vi "Spin In Circles Test (Test Turning PID).vi"() -> ()   [LabVIEW 2017]
uses:
  <vilib>/Platform/TimedLoop/XDataNode/XDataNode.xnode
  <vilib>/Platform/TimedLoop/XDataNode/nitl_modes.ctl
  <vilib>/Platform/TimedLoop/XDataNode/XDNodeRunTimeDep.lvlib
  <vilib>/Platform/TimedLoop/XDataNode/wakeup.ctl
  <vilib>/Platform/TimedLoop/XDataNode/timing_clust.ctl
  Globals/Pose.vi
  Globals/Motor Speed Multiplier.vi
panel:
  in  "Stop motors":bool=TRUE
  in  "Speed":T1={"\nMoving speed"=3.0889830508474576, "Turning speed limit"=1.0677966101694916} {"Turning speed limit" scale=0.0..4.0; "Moving speed" scale=0.0..1.0}
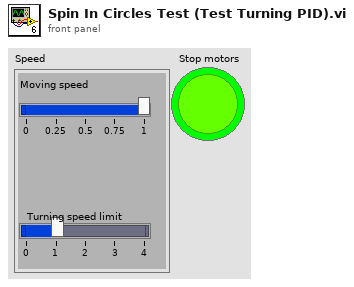
[diagram p1: front panel]
types:
  T1 = cluster{"\nMoving speed":dbl, "Turning speed limit":dbl}
  T2 = typedef "XDNodeRunTimeDep.lvlib/timing_clust.ctl" = cluster{"Expected End [f-1]":u64, "Actual End [f-1]":u64, "Finished Late? [f-1]":bool, "Expected End [i-1]":u64, "Actual End [i-1]":u64, "Finished Late? [i-1]":bool, "Expected Start [i]":u64, "Actual Start [i]":u64, "Expected Start [f]":u64, "Actual Start [f]":u64, "Source Name":string, "Structure Name":string, "Period":i64, "Deadline":i64, "Offset":i64, "Start":i64, "Priority":i32, "Timeout":i32, "Mode":T3, "Wakeup Reason":T4, "Error":errorcluster, "Source Type":string, "Secondary Source Type":string, "Global End Time":u64, "Global Start Time":u64, "Frame Duration":u64, "Iteration Duration":u64, "Assigned CPU":i32, "I/O Scan Engine Mode":u32}
  T3 = typedef "XDNodeRunTimeDep.lvlib/nitl_modes.ctl" = enum32{"No Change", "Process missed periods, maintain original phase", "Discard missed periods, maintain original phase", "Process missed periods, ignore original phase", "Discard missed periods, ignore original phase"}
  T4 = typedef "XDNodeRunTimeDep.lvlib/wakeup.ctl" = enum32{"Normal", "Aborted", "Asynchronous wakeup", "Timing source error", "Timed loop error", "Timeout"}
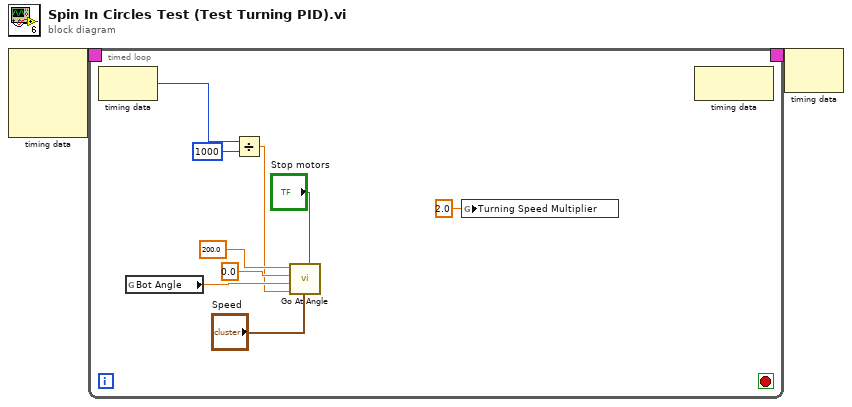
[diagram p0: block diagram]
diagram:
  n1 = node-c288() -> (w2:T2)  [unwired: 4 in]
  n2 = timed-loop {
    timing: w2 -> [_]
    timing-out: [_] -> w1
    stop <- _ stop-if-true
    n3 = node-c288() -> (w6:i64)  [unwired: 1 in]
    n4 = global read "Pose.vi" "Bot Angle"() -> (w9:dbl)
    n5 = Divide(x=w6, y=i64 1000) -> (x/y=w4:dbl)
    n6 = call "Go At Angle.vi"("Target Angle"=200.0 ("Target X (Relative)"), 1:0.0 ("Target Y (Relative)"), "Bot Angle"=w9, "dt"=w4, "Stop motors"="Stop motors", "Speed"="Speed") -> ()  [unwired: 5 in]
    n7 = global write "Motor Speed Multiplier.vi" "Turning Speed Multiplier"(2.0 ("Turning Speed Multiplier")) -> ()
    n8 = node-c288() -> ()  [unwired: 1 in, 1 out]
  }
  n9 = node-c288(w1) -> ()  [unwired: 1 out]
